vi "Write RequirementsMap.vi"(10 "Requirements":map{string, string}(c390), 11 "RequirementsFile in":refnum<class "RequirementsMap.lvclass">) -> (3 "RequirementsFile out":refnum<class "RequirementsMap.lvclass">)   [LabVIEW 2021, in "Bananas.lvlib" / "RequirementsMap.lvclass"]
uses:
  RequirementsMap.lvclass
  RequirementsMap.lvclass/RequirementsMap.ctl
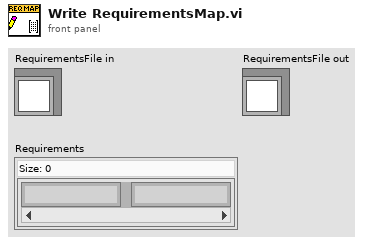
[diagram p1: front panel]
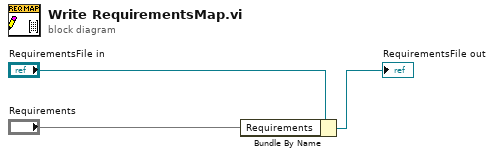
[diagram p0: block diagram]
diagram:
  n1 = Bundle By Name(cluster="RequirementsFile in", "Requirements"="Requirements") -> (→"RequirementsFile out":refnum<class "RequirementsMap.lvclass">)
